vi "Elevator Controller.vi"(8 "error in":errorcluster) -> ()   [LabVIEW 2017]
doc: "This VI executes continuously carrying out the current operation and responding to updates or new operations. It will often contain the timing or control code that is difficult to place directly in TeleOp. This VI generally opens all sensors and motors and isolates the rest of the robot code from knowing how the operations are carried out."
uses:
  <vilib>/Rock Robotics/WPI/Framework/Completion Status.ctl
  Elevator Setpoints.ctl
  Elevator Operations.ctl
  Private/Typedef/Elevator Settings.ctl
  Private/Typedef/Controller Data.ctl
  <vilib>/Rock Robotics/WPI/MotorControl/WPI_MotorControlDeviceRef.ctl
  <vilib>/Rock Robotics/WPI/MotorControl/WPI_MotorControlType.ctl
  <vilib>/Rock Robotics/SystemInterfaces/DIO/FPGA_DIOPWMChannel.ctl
  <vilib>/Rock Robotics/WPI/PWM/WPI_PWMDeadband.ctl
  <vilib>/Rock Robotics/SystemInterfaces/DIO/FPGA_DIOChannel.ctl
  <vilib>/Rock Robotics/WPI/Encoder/WPI_EncoderDevRef.ctl
  <vilib>/Rock Robotics/SystemInterfaces/Encoder/FPGA_EncoderIdx.ctl
  <vilib>/Rock Robotics/SystemInterfaces/Counter/FPGA_CounterCtrSystemIndex.ctl
  <vilib>/Rock Robotics/WPI/Encoder/WPI_EncoderType.ctl
  <vilib>/Rock Robotics/WPI/DigitalInput/WPI_DigitalInputDevRef.ctl
panel:
  in  "Settings":T1={"output range"={"output high"=1.0, "output low"=-0.8}, "min speed"=0.05, "homing speed"=0.05, "Position Max"=68.0, "PIDF gains"={"Kp"=0.2, "Ki"=0.0, "Kd"=0.2, "Kf"=0.0}, "gravity"=0.03, "Rate Limit in/sec"=30.0} {"Rate Limit in/sec" format="%#_13g"; "gravity" format="%#_13g"; "PIDF gains"."Kf" format="%.5f"; "PIDF gains"."Kd" format="%.3f"; "PIDF gains"."Ki" format="%.3f"; "PIDF gains"."Kp" format="%.3f"; "Position Max" format="%#_13g"; "homing speed" format="%#_13g"; "min speed" format="%#_13g"; "output range"."output low" format="%.2f"; "output range"."output high" format="%.2f"}
  out "Sensor":dbl
  out "Switches":T2
  out "Graph Out":T3(graph)
  in  "Interactive Values":T4
  out "Current\nCmd":string
  in  "Buttons":cluster{"Execute Cmd":bool, "Abort Cmd":bool}
  out "Command Timing":cluster{"Start Time (ms)":u32, "Iterations":i32}
  out "Status":T6
  # "Interactive Command: You may fill in the settings for a command\nand schedule it with the Execute button. You can observe and abort\nany command while fine tuning the code for the controller."
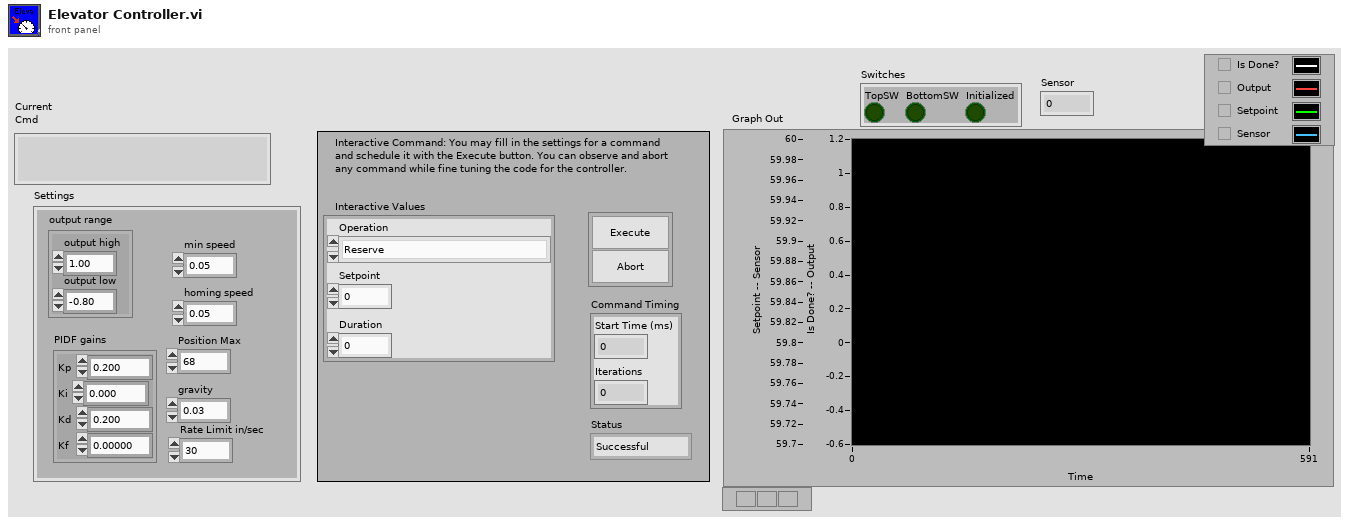
[diagram p1: front panel]
types:
  T1 = typedef "Elevator Settings.ctl" = cluster{"output range":cluster{"output high":dbl, "output low":dbl}, "min speed":dbl, "homing speed":dbl, "Position Max":dbl, "PIDF gains":cluster{"Kp":dbl, "Ki":dbl, "Kd":dbl, "Kf":dbl}, "gravity":dbl, "Rate Limit in/sec":dbl}
  T2 = cluster{"TopSW":bool, "BottomSW":bool, "Initialized":bool}
  T3 = cluster{i16, dbl, "Setpoint":dbl, "Distance":dbl}
  T4 = typedef "Elevator Setpoints.ctl" = cluster{"Operation":T5, "Setpoint":dbl, "Duration":dbl}
  T5 = typedef "Elevator Operations.ctl" = enum16{"Reserve", "Read Current", "Immediate", "Stop", "Switch", "Scale", "Home", "Go to Position"}
  T6 = typedef "Completion Status.ctl" = enum16{"Successful", "Aborted", "Incomplete"}
  T7 = typedef "Controller Data.ctl" = cluster{"Setpoint":dbl, "Output":dbl, "DriveMotor1":T8, "Encoder":T13, "DriveMotor2":T8, "Top SW":T17, "Bottom SW":T17, "Is Done Moving?":bool}
  T8 = typedef "WPI_MotorControlDeviceRef.ctl" = cluster{"DeviceStatus":errorcluster, "Type":T9, "PWM":cluster{"PWM Channel":T10, "DeadBand":T11}, "CAN":cluster{"Device Number":u8, "SetOutput VI Ref":variant, "GetOutput VI Ref":variant, "Enable VI Ref":variant, "Disable VI Ref":variant, "Data":variant}, "Invert":bool, "DIO PWM":cluster{"PWM \"Enable\" Channel":T10, "DIOChannel":T12, "PWM Rate":dbl}}
  T9 = typedef "WPI_MotorControlType.ctl" = enum16{"PWM", "CAN", "DIO PWM"}
  T10 = typedef "FPGA_DIOPWMChannel.ctl" = enum8{"PWM 0", "PWM 1", "PWM 2", "PWM 3", "PWM 4", "PWM 5", "PWM 6", "PWM 7", "PWM 8", "PWM 9", "PWM MXP 0", "PWM MXP 1", "PWM MXP 2", "PWM MXP 3", "PWM MXP 4", "PWM MXP 5", "PWM MXP 6", "PWM MXP 7", "PWM MXP 8", "PWM MXP 9", "Invalid"}
  T11 = typedef "WPI_PWMDeadband.ctl" = cluster{"Name":string, "maxPositivePwm":i32, "minPositivePwm":i32, "centerPwm":i32, "maxNegativePwm":i32, "minNegativePwm":i32, "angularRange":u16}
  T12 = typedef "FPGA_DIOChannel.ctl" = enum8{"DIO 0", "DIO 1", "DIO 2", "DIO 3", "DIO 4", "DIO 5", "DIO 6", "DIO 7", "DIO 8", "DIO 9", "DIO MXP 0", "DIO MXP 1", "DIO MXP 2", "DIO MXP 3", "DIO MXP 4", "DIO MXP 5", "DIO MXP 6", "DIO MXP 7", "DIO MXP 8", "DIO MXP 9", "DIO MXP 10", "DIO MXP 11", "DIO MXP 12", "DIO MXP 13", "DIO MXP 14", "DIO MXP 15", "SPI Port CS1", "SPI Port CS2", "SPI Port CS3", "SPI Port MISO", "SPI Port MOSI", "Invalid"}
  T13 = typedef "WPI_EncoderDevRef.ctl" = cluster{"DevStatus":errorcluster, "EncoderIndex":T14, "CounterIndex":T15, "DistancePerCount":dbl, "Decoding Type":T16}
  T14 = typedef "FPGA_EncoderIdx.ctl" = enum8{"Enc 0", "Enc 1", "Enc 2", "Enc 3", "Enc 4", "Enc 5", "Enc 6", "Enc 7", "Invalid"}
  T15 = typedef "FPGA_CounterCtrSystemIndex.ctl" = enum8{"Ctr 0", "Ctr 1", "Ctr 2", "Ctr 3", "Ctr 4", "Ctr 5", "Ctr 6", "Ctr 7", "Invalid"}
  T16 = typedef "WPI_EncoderType.ctl" = enum16{"1x", "2x", "4x"}
  T17 = typedef "WPI_DigitalInputDevRef.ctl" = cluster{"DevStatus":errorcluster, "DIO Channel":T12}
  T18 = typedef "Command Status Info.ctl" = cluster{"Name":string, "Status":T6, "notifier out":T19}
  T19 = typedef "Completion Notifier.ctl" = refnum<notifier>
  T20 = cluster{"Current Command":T4, "Command Timing":cluster{"Start Time (ms)":u32, "Iterations":i32}, "Command Arguments":cluster{"Command Info":T18, "Description":string, "Default Command":T4, "queue out":refnum<queue>, "Subsystem Name":string}}
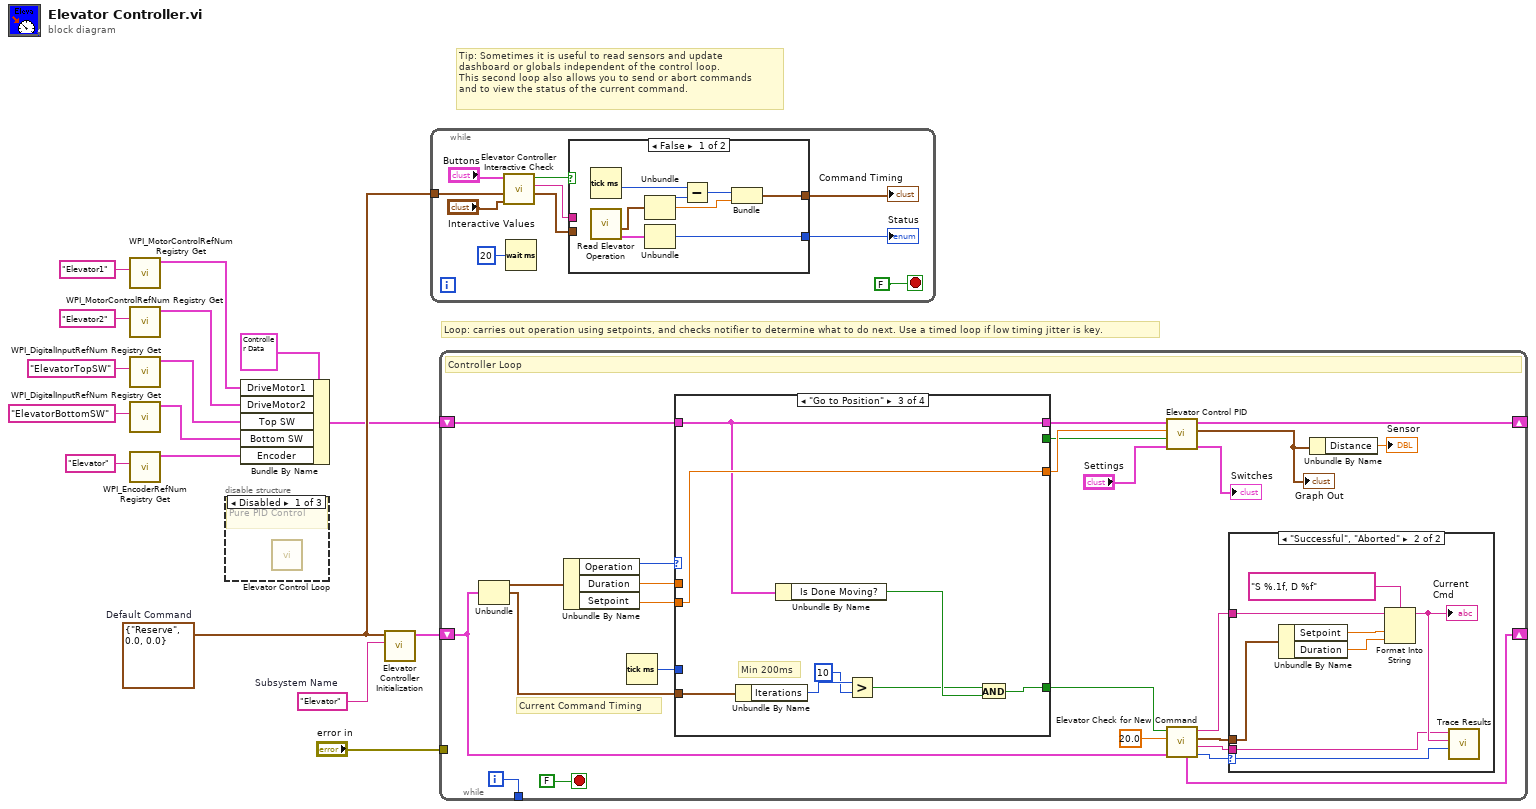
[diagram p0: block diagram]
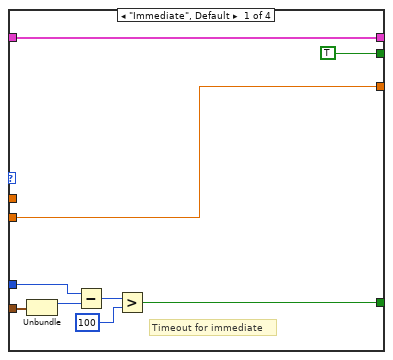
[diagram p2: hidden frame]
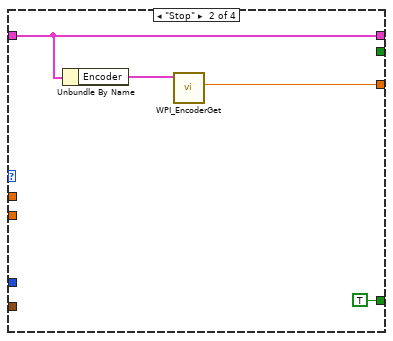
[diagram p3: hidden frame]
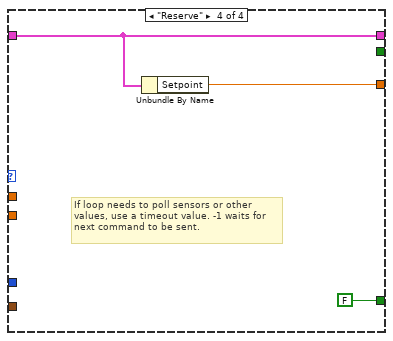
[diagram p4: hidden frame]
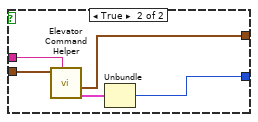
[diagram p6: hidden frame]
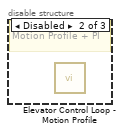
[diagram p7: hidden frame]
diagram:
  w14 = T4 {"Operation"=enum."Reserve", "Setpoint"=0.0, "Duration"=0.0}  # Default Command
  w15 = "Elevator"  # Subsystem Name
  # "Tip: Sometimes it is useful to read sensors and update\ndashboard or globals independent of the control loop.\nThis second loop also allows you to send or abort commands\nand to view the status of the current command."
  # "Loop: carries out operation using setpoints, and checks notifier to determine what to do next. Use a timed loop if low timing jitter is key."
  n1 = call <vilib>:"WPI_MotorControlRefNum Registry Get.vi"("refnum name"="Elevator1") -> ("MotorControlDevRef"=w6:T8)  [unwired: 9 in, 1 out]
  n2 = call <vilib>:"WPI_MotorControlRefNum Registry Get.vi"("refnum name"="Elevator2") -> ("MotorControlDevRef"=w5:T8)  [unwired: 9 in, 1 out]
  n3 = call <vilib>:"WPI_DigitalInputRefNum Registry Get.vi"("refnum name"="ElevatorTopSW") -> ("DigitalInputDevRef"=w4:T17)  [unwired: 9 in, 1 out]
  n4 = call <vilib>:"WPI_DigitalInputRefNum Registry Get.vi"("refnum name"="ElevatorBottomSW") -> ("DigitalInputDevRef"=w3:T17)  [unwired: 9 in, 1 out]
  n5 = call <vilib>:"WPI_EncoderRefNum Registry Get.vi"("refnum name"="Elevator") -> ("EncoderDevRef"=w2:T13)  [unwired: 9 in, 1 out]
  n6 = disable-structure shown="Disabled" {
    frame Disabled {
      # "Pure PID Control"
      n7 = call "Elevator Control Loop.vi"() -> ()  [unwired: 12 in]
    }
    frame Disabled {
      # "Motion Profile + PI"
      n8 = call "Elevator Control Loop - Motion Profile.vi"() -> ()  [unwired: 12 in]
    }
    frame Enabled {
      # "OLD"
    }
  }
  n9 = Bundle By Name(cluster=T7 {"Setpoint"=0.0, "Output"=0.0, "DriveMotor1"={"DeviceStatus"={"status"=FALSE, "code"=0, "source"=""}, "Type"=enum."PWM", "PWM"={"PWM Channel"=enum."Invalid", "DeadBand"={"Name"="", "maxPositivePwm"=0, "minPositivePwm"=0, "centerPwm"=0, "maxNegativePwm"=0, "minNegativePwm"=0, "angularRange"=0}}, "CAN"={"Device Number"=0, "SetOutput VI Ref"=variant(enum8{"Percent VBus", "Current", "Speed", "Position", "Voltage"} enum."Percent VBus"), "GetOutput VI Ref"=variant(refnum<k1> refnum), "Enable VI Ref"=variant(dbl 12.0), "Disable VI Ref"=variant(enum8{"Percent VBus", "Speed", "Position", "Slave", "Unchanged / Invalid"} enum."Percent VBus"), "Data"=variant(enum16{"Controller 1"} enum."Controller 1")}, "Invert"=FALSE, "DIO PWM"={"PWM \"Enable\" Channel"=enum."Invalid", "DIOChannel"=enum."Invalid", "PWM Rate"=0.0}}, "Encoder"={"DevStatus"={"status"=FALSE, "code"=0, "source"=""}, "EncoderIndex"=enum."Invalid", "CounterIndex"=enum."Invalid", "DistancePerCount"=1.0, "Decoding Type"=enum."4x"}, "DriveMotor2"={"DeviceStatus"={"status"=FALSE, "code"=0, "source"=""}, "Type"=enum."PWM", "PWM"={"PWM Channel"=enum."Invalid", "DeadBand"={"Name"="", "maxPositivePwm"=0, "minPositivePwm"=0, "centerPwm"=0, "maxNegativePwm"=0, "minNegativePwm"=0, "angularRange"=0}}, "CAN"={"Device Number"=0, "SetOutput VI Ref"=variant(enum8{"Percent VBus", "Current", "Speed", "Position", "Voltage"} enum."Percent VBus"), "GetOutput VI Ref"=variant(refnum<k1> refnum), "Enable VI Ref"=variant(dbl 12.0), "Disable VI Ref"=variant(enum8{"Percent VBus", "Speed", "Position", "Slave", "Unchanged / Invalid"} enum."Percent VBus"), "Data"=variant(enum16{"Controller 1"} enum."Controller 1")}, "Invert"=FALSE, "DIO PWM"={"PWM \"Enable\" Channel"=enum."Invalid", "DIOChannel"=enum."Invalid", "PWM Rate"=0.0}}, "Top SW"={"DevStatus"={"status"=FALSE, "code"=0, "source"=""}, "DIO Channel"=enum."Invalid"}, "Bottom SW"={"DevStatus"={"status"=FALSE, "code"=0, "source"=""}, "DIO Channel"=enum."Invalid"}, "Is Done Moving?"=FALSE}, "DriveMotor1"=w6, "DriveMotor2"=w5, "Top SW"=w4, "Bottom SW"=w3, "Encoder"=w2) -> (w1:T7)
  n10 = call "Elevator Controller Initialization.vi"("Subsystem Name"=w15, "Default Command"=w14) -> ("Current Command"=w13:T20)  [unwired: 9 in]
  n11 = while {
    tunnel: w14 -> [w23]
    stop <- FALSE stop-if-true
    n12 = call "Elevator Controller Interactive Check.vi"("Interactive Command in"="Interactive Values", "Default Command"=w23, "Buttons"="Buttons") -> ("Interactive Command out"=w20:T4, "Trace String"=w21:string, "Schedule"=w22:bool)  [unwired: 6 in]
    n13 = Wait (ms)(milliseconds to wait=u32 20) -> ()  [unwired: 1 out]
    n14 = case shown="False" w22 {
      tunnel: [w34 w39] -> w19
      tunnel: w20 -> [_ w37]
      tunnel: [w30 w35] -> w18
      tunnel: w21 -> [_ w38]
      frame False {
        n15 = Tick Count (ms)() -> (millisecond timer value=w29:u32)
        n16 = call "Read Elevator Operation.vi"() -> ("Command Info"=w27:T18, "SubSystem Data"=w28:T4)  [unwired: 9 in, 1 out]
        n17 = Unbundle(w28) -> ("Operation"=w33:T5, "Setpoint"=w31:dbl)  [unwired: 1 out]
        n18 = Unbundle(w27) -> ("Status"=w34:T6)  [unwired: 2 out]
        n19 = Subtract(x=w29, y=w33) -> (x-y=w32:u32)
        n20 = Bundle(w32, "Setpoint"=w31) -> (w30:cluster{u32, "Setpoint":dbl})  [unwired: 1 in]
      }
      frame True {
        n21 = call "Elevator Command Helper.vi"("Description"=w38, "SubSystem Data"=w37) -> ("Command Info Out"=w36:T18, "Command Timing"=w35:cluster{"Start Time (ms)":u32, "Iterations":i32})  [unwired: 7 in, 1 out]
        n22 = Unbundle(w36) -> ("Status"=w39:T6)  [unwired: 2 out]
      }
    }
    "Status" <- w19
    "Command Timing" <- w18
  }
  n23 = while {
    shift-right: [w56] -> _
    shift-left: w13 -> [w50]
    tunnel: [w63] -> _
    tunnel: "error in" -> [_]
    shift-right: [w47] -> _
    shift-left: w1 -> [w49]
    i -> [w63]
    stop <- FALSE stop-if-true
    # "Current Command Timing"
    # "Controller Loop"
    n24 = Unbundle(w50) -> ("Current Command"=w62:T4, "Command Timing"=w58:cluster{"Start Time (ms)":u32, "Iterations":i32})  [unwired: 1 out]
    n25 = Unbundle By Name(w62) -> ("Operation"=w61:T5, "Duration"=w60:dbl, "Setpoint"=w57:dbl)
    n26 = Tick Count (ms)() -> (millisecond timer value=w59:u32)
    n27 = case shown="\"Go to Position\"" w61 {
      tunnel: [w68 TRUE ("ignore previous (F)") w79 FALSE ("ignore previous (F)")] -> w55
      tunnel: w58 -> [w70 _ w82 _]
      tunnel: w60 -> [_ _ _ _]
      tunnel: w59 -> [w69 _ _ _]
      tunnel: w57 -> [w65 _ w85 _]
      tunnel: w49 -> [w67 w77 w84 w87]
      tunnel: [w67 w77 w84 w87] -> w48
      tunnel: [w65 w74 w85 w86] -> w46
      tunnel: [TRUE _ _ _] -> w45
      frame "Immediate", Default {
        # "Timeout for immediate"
        n28 = Unbundle(w70) -> ("Start Time (ms)"=w73:u32)  [unwired: 1 out]
        n29 = Subtract(x=w69, y=w73) -> (x-y=w72:u32)
        n30 = Greater?(x=w72, y=u8 100 ("Left Motor")) -> (0:w68:bool)
      }
      frame "Stop" {
        n31 = Unbundle By Name(w77) -> ("Encoder"=w75:T13)
        n32 = call <vilib>:"WPI_EncoderGet.vi"("EncoderDevRef"=w75) -> ("Distance"=w74:dbl)  [unwired: 5 in, 5 out]
      }
      frame "Go to Position" {
        # "Min 200ms"
        n33 = Unbundle By Name(w82) -> ("Iterations"=w81:i32)
        n34 = Unbundle By Name(w84) -> ("Is Done Moving?"=w83:bool)
        n35 = Greater?(x=w81, y=10 ("x")) -> (0:w78:bool)
        n36 = And(x=w78, y=w83) -> (x .and. y?=w79:bool)
      }
      frame "Reserve" {
        # "If loop needs to poll sensors or other\nvalues, use a timeout value. -1 waits for\nnext command to be sent."
        n37 = Unbundle By Name(w87) -> ("Setpoint"=w86:dbl)
      }
    }
    n38 = call "Elevator Control PID.vi"("Settings"="Settings", "Manual"=w45, "Setpoint"=w46, "Controller In"=w48) -> ("Switches"=→"Switches":T2, "Graph Out"=w42:T3, "Controller out"=w47:T7)  [unwired: 4 in, 1 out]
    "Graph Out" <- w42
    n39 = call "Elevator Check for New Command.vi"("Current Command"=w50, "Wait time (ms)"=20.0, "Finished?"=w55) -> ("Completion"=w51:T6, "Subsystem Name"=w52:string, "Current Command"=w53:T4, "Initial Trace String"=w54:string, "NextCommand"=w56:T20)  [unwired: 4 in]
    n40 = case shown="\"Successful\", \"Aborted\"" w51 {
      selector: w51 -> [_ w89]
      tunnel: w54 -> [_ w93]
      tunnel: w53 -> [_ w94]
      tunnel: w52 -> [_ w90]
      frame "Incomplete", Default {
        # "Continuing current command"
      }
      frame "Successful", "Aborted" {
        # "Report and setup for next command"
        n41 = Unbundle By Name(w94) -> ("Setpoint"=w96:dbl, "Duration"=w91:dbl)
        n42 = Format Into String(format string="S %.1f, D %f", initial string=w93, w96, w91) -> (resulting string=w92:string)  [unwired: 1 in, 1 out]
        "Current\nCmd" <- w92
        n43 = call <vilib>:"Trace Results.vi"("Status of previous command"=w89, "Description"=w92, "Subsystem"=w90) -> ()  [unwired: 9 in]
      }
    }
    n44 = Unbundle By Name(w42) -> ("Distance"=→"Sensor":dbl)
  }
